vi "requestSlitPosition.vi"(8 "error in (no error)":errorcluster, 10 "SlitType":T1, 11 "MonoCommunicator in":refnum<class "MonoCommunicator.lvclass">) -> (0 "error out":errorcluster, 3 "MonoCommunicator out":refnum<class "MonoCommunicator.lvclass">)   [LabVIEW 2016, in "MonoCommunicator.lvclass"]
uses:
  MonoCommunicator.lvclass
  Typedefs/SlitType.ctl
  MonoCommunicator.lvclass/MonoCommunicator.ctl
  MonoPubSubData/MonoPubSubData.lvclass/MonoPubSubData.ctl
  MonoPubSubData/MonoPubSubData.lvclass
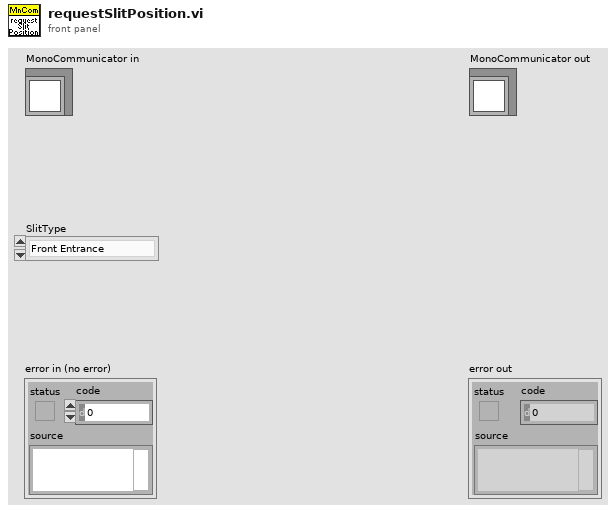
[diagram p1: front panel]
types:
  T1 = typedef "SlitType.ctl" = enum16{"Front Entrance", "Side Entrance", "Front Exit", "Side Exit", "First Intermediate", "Second Intermediate"}
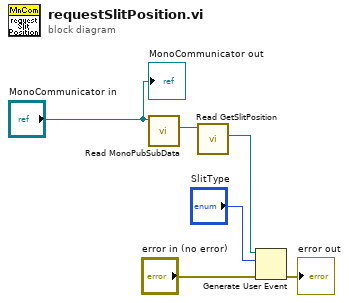
[diagram p0: block diagram]
diagram:
  n1 = call "Read MonoPubSubData.vi"("MonoCommunicator in"="MonoCommunicator in") -> ("MonoPubSubData.lvclass"=w5:refnum<class "MonoPubSubData.lvclass">)  [unwired: 8 in, 2 out]
  n2 = call "Read GetSlitPosition.vi"("MonoPubSubData in"=w5) -> ("GetSlitPosition"=w4:refnum<user-event>)  [unwired: 8 in, 2 out]
  n3 = Generate User Event(user event=w4, event data cluster="SlitType", error in="error in (no error)") -> (error out=→"error out":errorcluster)  [unwired: 1 in, 1 out]
  "MonoCommunicator out" <- "MonoCommunicator in"
